vi "Do.vi"(8 "error in":errorcluster, 10 "Actor in":refnum<class "Actor.lvclass">, 11 "File Data Message":refnum<class "File Data Message.lvclass">) -> (0 "error out":errorcluster, 2 "Actor out":refnum<class "Actor.lvclass">)   [LabVIEW 2014, in "File Library.lvlib" / "File Data Message.lvclass"]
doc: "(<B>Filename</B>: Actor Framework.lvlib:Message.lvclass:Do.vi)\n\nDefines what a message does when it is received by an actor. Generally, a message instructs an actor to invoke one of its methods. By default, this method does nothing. A child class must override it to define behavior. Create a child class by using the Actor Framework Message Maker dialog box."
uses:
  File Data Message.lvclass
  <vilib>/ActorFramework/Actor/Actor.lvclass
  File Data Message.lvclass/File Data Message.ctl
  File Actor.lvclass
  SuperActor/Ex Nested.lvclass/Ex Nested.ctl
  File Actor.lvclass/File Actor.ctl
  Abstract/Exe Write/Exe Write.lvclass/Exe Write.ctl
  SuperActor/Read Log Session.vi
  Read Exe File Write.vi
  Read Exe Write.vi
  Abstract/Exe Write/Write Data.vi
  Abstract/Exe Write/Exe Write.lvclass
  reusable/Command/Command.lvclass
  <userlib>/_Session Fwk/Session - Root.lvclass
  reusable/Session APIs/Session Log/System Log.lvclass
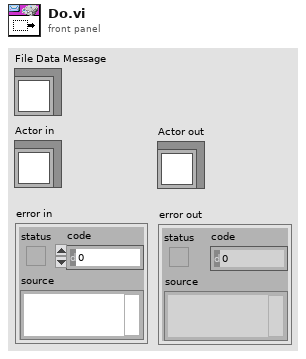
[diagram p1: front panel]
types:
  T1 = typedef "Session - Root.lvclass/Session Handle.ctl" = refnum<data-value>
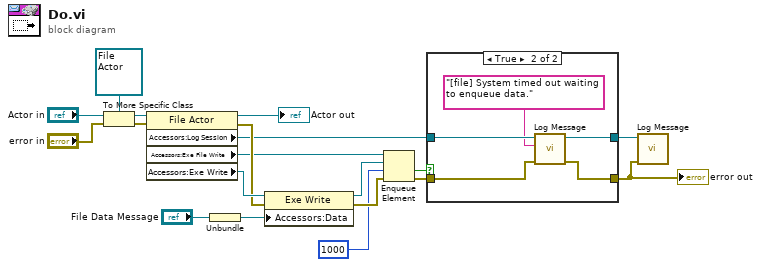
[diagram p0: block diagram]
diagram:
  n1 = To More Specific Class(target class=refnum<class "File Actor.lvclass"> refnum ("File Library.lvlib:File Actor"), reference="Actor in", error in="error in") -> (specific class reference=w15:refnum<class "File Actor.lvclass">, error out=w14:errorcluster)
  n2 = property class="File Actor"(reference=w15, error in=w14) -> (reference out=→"Actor out":refnum<class "File Actor.lvclass">, error out=w7:errorcluster, "Accessors:Log Session"=w1:T1, "Accessors:Exe File Write"=w2:refnum<queue>, "Accessors:Exe Write"=w10:refnum<class "Exe Write.lvclass">)
  n3 = Unbundle("File Data Message") -> (w9:refnum<class "Data.lvclass">)
  n4 = property class="Exe Write"(reference=w10, error in=w7, "Accessors:Data"=w9) -> (reference out=w8:refnum<class "Exe Write.lvclass">, error out=w6:errorcluster)
  n5 = Enqueue Element(queue=w2, element=w8, timeout in ms (-1)=1000, error in (no error)=w6) -> (timed out?=w4:bool, error out=w5:errorcluster)  [unwired: 1 out]
  n6 = case shown="True" w4 {
    tunnel: w5 -> [w21 w23]
    tunnel: w1 -> [w20 w26]
    tunnel: [w21 w22] -> w12
    tunnel: [w20 w24] -> w13
    frame False {
    }
    frame True {
      n7 = call "Log Message.vi"("error in"=w23, "MSG In"="[file] System timed out waiting to enqueue data.", "session in"=w26) -> ("error out"=w22:errorcluster, "session out"=w24:T1)  [unwired: 7 in]
    }
  }
  "error out" <- w12
  n8 = call "Log Message.vi"("error in"=w12, "session in"=w13) -> ()  [unwired: 8 in, 2 out]
